vi "Endpoint_Connected_For_P3AT.vi"(8 "error in (no error)":errorcluster, 10 "Endpoint Enqueuer":refnum<class "Message Enqueuer.lvclass">, 11 "Remote Endpoint P3AT Actor.lvlib:Remote Endpoint P3AT.lvclass in":refnum<class "RemoteP3AT.lvclass">) -> (0 "error out":errorcluster, 3 "Remote Endpoint P3AT Actor.lvlib:Remote Endpoint P3AT.lvclass out":refnum<class "RemoteP3AT.lvclass">)   [LabVIEW 2014]
uses:
  <vilib>/ActorFramework/Message Enqueuer/Message Enqueuer.lvclass
  RemoteP3AT.lvclass
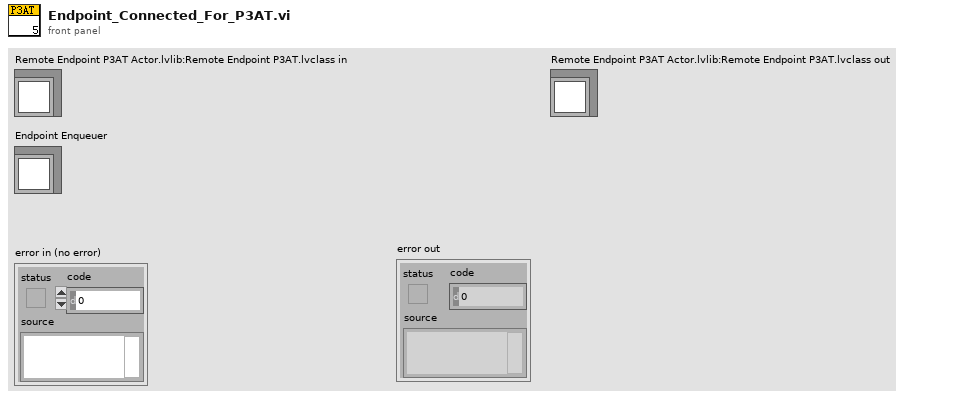
[diagram p1: front panel]
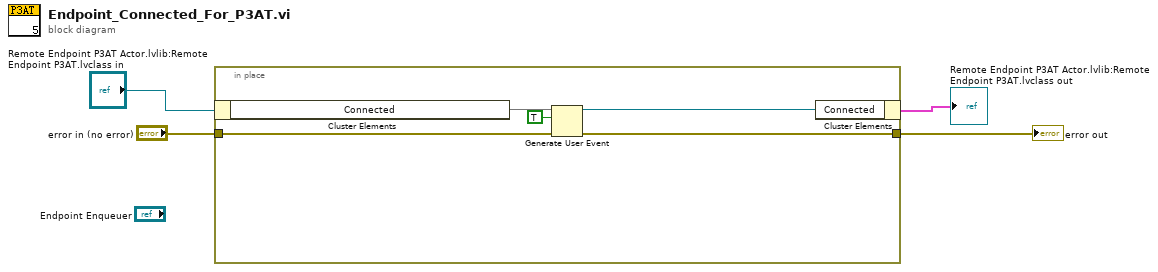
[diagram p0: block diagram]
diagram:
  n1 = in-place {
    in-place-border: "error in (no error)" -> [w7]
    in-place-border: [w6] -> w3
    n2 = in-place-cluster #1("Remote Endpoint P3AT Actor.lvlib:Remote Endpoint P3AT.lvclass in") -> ("Connected"=w9)
    n3 = Generate User Event(user event=w9, event data cluster=TRUE ("event data"), error in=w7) -> (user event out=w8:refnum<user-event>, error out=w6:errorcluster)  [unwired: 1 in]
    n4 = in-place-cluster #1("Connected"=w8) -> (→"Remote Endpoint P3AT Actor.lvlib:Remote Endpoint P3AT.lvclass out":cluster{})
  }
  "error out" <- w3
